vi "Terminal-Alert-Trigger.vi"(8 "error in (no error)":errorcluster caption="错误输入（无错误）", 10 "报警信息":T1, 11 "是否触发(T)":bool=TRUE) -> (0 "error out":errorcluster caption="错误输出")   [LabVIEW 2014]
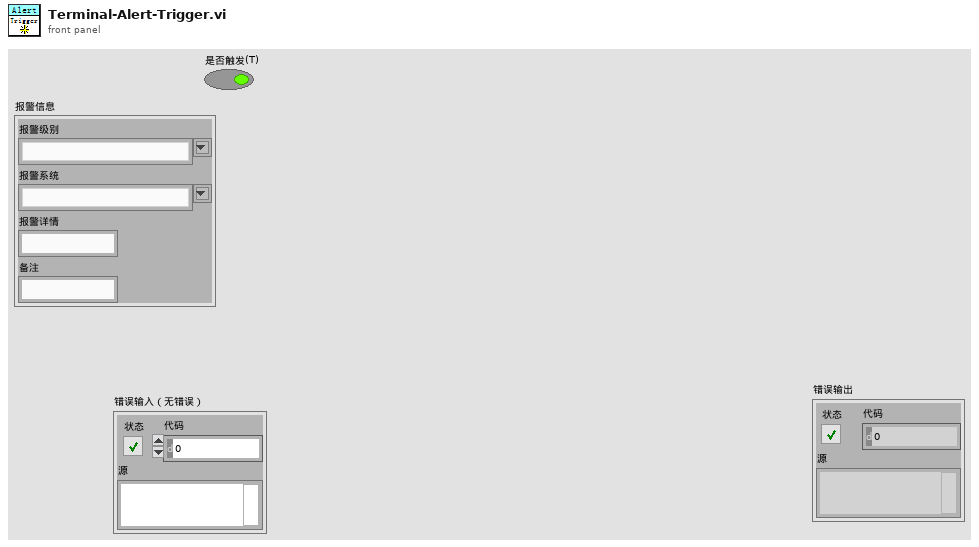
[diagram p1: front panel]
types:
  T1 = cluster{"报警级别":string, "报警系统":string, "报警详情":string, "备注":string}
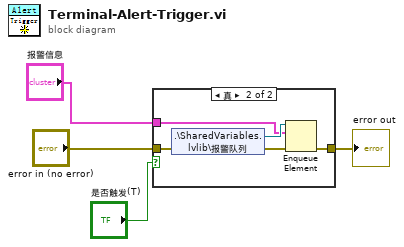
[diagram p0: block diagram]
diagram:
  n1 = case shown="真" "是否触发(T)" {
    tunnel: "error in (no error)" -> [w5 w8]
    tunnel: [w5 w7] -> w2
    tunnel: "报警信息" -> [_ w6]
    frame False {
    }
    frame True {
      n2 = shared-variable ".\\SharedVariables.lvlib\\报警队列"(error in=w8) -> (w10:refnum<queue>, error out=w9:errorcluster)
      n3 = Enqueue Element(queue=w10, element=w6, error in (no error)=w9) -> (error out=w7:errorcluster)  [unwired: 1 in, 2 out]
    }
  }
  "error out" <- w2
